vi "Start Lockin Sweep.vi"(8 "error in (no error)":errorcluster, 11 "MeasurementSMO in":refnum<class "MeasurementSMO.lvclass">) -> (0 "error out":errorcluster, 3 "MeasurementSMO out":refnum<class "MeasurementSMO.lvclass">)   [LabVIEW 2019, in "MeasurementSMO.lvclass"]
uses:
  MeasurementSMO.lvclass
  MeasurementSMO.lvclass/MeasurementSMO.ctl
  f5997dcf-fa52-409d-918b-a65a3faecfae.vi
  f5997dcf-fa52-409d-918b-a65a3faecfae.vi/ff40df25-0e41-4205-825d-56c19dc320b6.vi
  <vilib>/Utility/Debug Log/Display.vi
  <userlib>/LevyLab/Lockin-Multichannel/Instrument.Lockin/Instrument.Lockin.lvclass
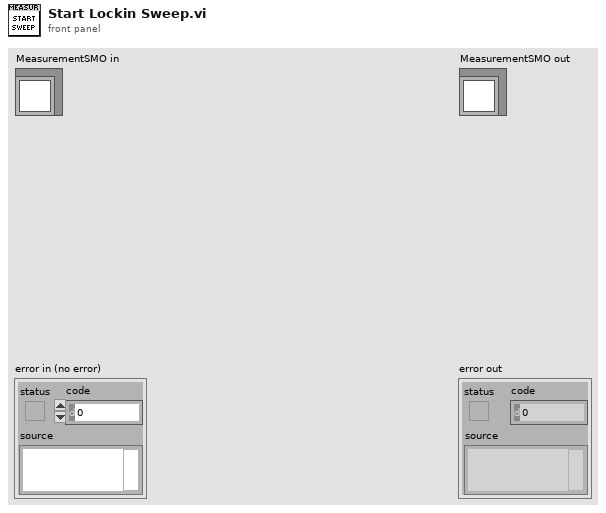
[diagram p1: front panel]
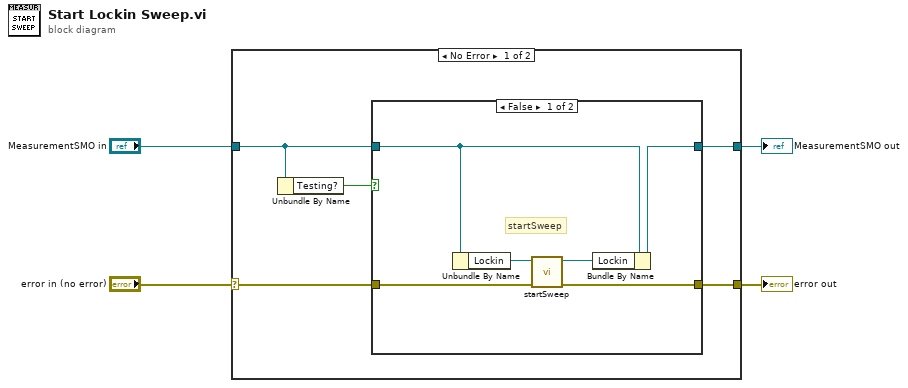
[diagram p0: block diagram]
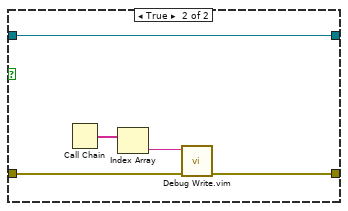
[diagram p2: hidden frame]
diagram:
  n1 = case shown="No Error" "error in (no error)" {
    selector: "error in (no error)" -> [w5 w22]
    tunnel: [w6 w22] -> w3
    tunnel: [w7 w21] -> w1
    tunnel: "MeasurementSMO in" -> [w8 w21]
    frame No Error {
      n2 = Unbundle By Name(w8) -> ("Testing?"=w9:bool)
      n3 = case shown="False" w9 {
        tunnel: w8 -> [w14 w20]
        tunnel: [w15 w20] -> w7
        tunnel: [w10 w19] -> w6
        tunnel: w5 -> [w11 w18]
        frame False {
          # "startSweep"
          n4 = Unbundle By Name(w14) -> ("Lockin"=w13:refnum<class "Instrument.Lockin.lvclass">)
          n5 = call <userlib>:"startSweep.vi"("error in (no error)"=w11, "Instrument.Lockin in"=w13) -> ("error out"=w10:errorcluster, "Instrument.Lockin out"=w12:refnum<class "Instrument.Lockin.lvclass">)  [unwired: 8 in]
          n6 = Bundle By Name(cluster=w14, "Lockin"=w12) -> (w15:refnum<class "MeasurementSMO.lvclass">)
        }
        frame True {
          n7 = Call Chain() -> (call chain=w16:string[])
          n8 = Index Array(array=w16) -> (element=w17:string)  [unwired: 1 in]
          n9 = call "Debug Write.vim"("error in (no error)"=w18, "value"=w17) -> ("error out"=w19:errorcluster)  [unwired: 9 in]
        }
      }
    }
    frame Error {
    }
  }
  "error out" <- w3
  "MeasurementSMO out" <- w1
